vi "ACC_LabVIEW_Read_Example.vi"() -> ()   [LabVIEW 2014, in "ACC_LabVIEW.lvlib"]
doc: "Example for using the \"read\" method."
uses:
  ACC_LabVIEW.lvlib
  DataConverter/Acc2LabVIEWData_String.vi
  DataConverter/Acc2LabVIEWData_SWord.vi
panel:
  out "EFICD":T1
  out "LV_TimeStamp":T2
  out "Device Properties":T3(array[cluster])
  out "error out":errorcluster
  in  "#of expected Elements in \"Acc_Data_Out\"":u32=200
  in  "Propname[20]":string="PROPDESC"
  in  "Nomenklatur[6]":string="K4XCS012"
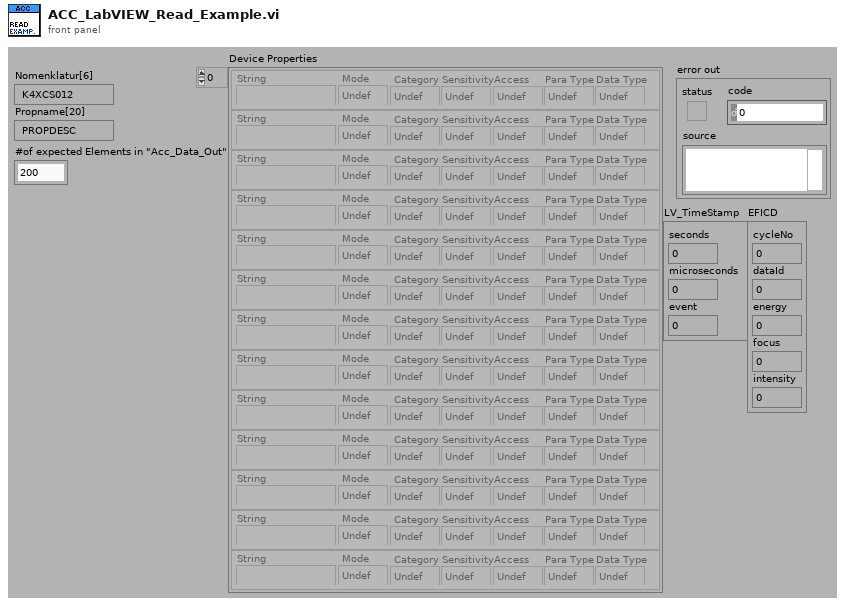
[diagram p1: front panel]
types:
  T1 = cluster{"cycleNo":u32, "dataId":u32, "energy":u32, "focus":u32, "intensity":u32}
  T2 = cluster{"seconds":u32, "microseconds":u32, "event":u32}
  T3 = cluster{"String":string, " Mode":enum16{"Undef", "Read", "Write", "Call"}, " Category":enum16{"Undef", "Master", "Slave"}, "Sensitivity":enum16{"Undef", "All", "VrtAcc", "None"}, "Access":enum16{"Undef", "Free", "Device", "System", "Critical"}, "Para Type":enum16{"Undef", "BitSet8", "BitSet16", "BitSet32", "Integer16", "Integer32", "Fix16", "Fix32", "RealF", "Real32", "Integer8", "RealG", "Structure", "BitSet64", "Integer64", "Real64"}, "Data Type":enum16{"Undef", "BitSet8", "BitSet16", "BitSet32", "Integer16", "Integer32", "Fix16", "Fix32", "RealF", "Real32", "Integer8", "RealG", "Structure", "BitSet64", "Integer64", "Real64"}}[]
  T4 = typedef "ACC_LabVIEW.lvlib/ACC_LabVIEW_Container.ctl" = cluster{"Data Type":T5, "String":string, "Double":dbl}
  T5 = typedef "ACC_LabVIEW.lvlib/ACC_LabVIEW_DataTypes.ctl" = enum16{"SByte (8Bit Int signed)", "UByte (8Bit int unsigned)", "SWord (16Bit Int signed)", "UWord (16Bit Int unsigned)", "SLong (32Bit Int signed)", "ULong (32Bit Int unsigned)", "Float32 (float)", "Float64 (double)", "String"}
  T6 = cluster{"Value":string, "Value":i16, "Value":i16, "Value":i16, "Value":i16, "Value":i16, "Value":i16}
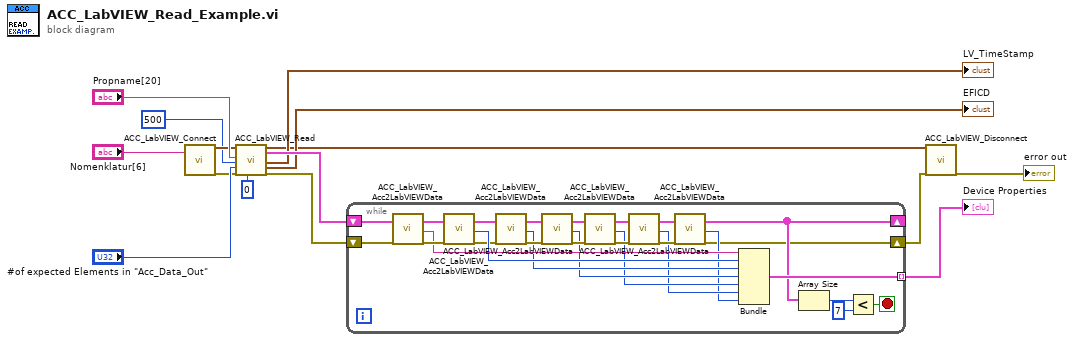
[diagram p0: block diagram]
diagram:
  n1 = call "ACC_LabVIEW_Connect.vi"("Nomenklatur"="Nomenklatur[6]") -> ("DeviceReferenceOut"=w5:cluster{"ID":u32}, "error out"=w8:errorcluster)  [unwired: 17 in]
  n2 = call "ACC_LabVIEW_Read.vi"("DeviceReferenceIn"=w5, "Propname"="Propname[20]", "return data string buffer size (Byte)"=u32 500 ("return strings buffer size (Byte)"), "#of expected Elements in \"Acc_Data_Out\""="#of expected Elements in \"Acc_Data_Out\"", "error in (no error)"=w8, "VirtAcc"=0) -> ("DeviceReferenceOut"=w7:cluster{"ID":u32}, "Acc_Data_Out"=w12:T4[], "LV_TimeStamp"=→"LV_TimeStamp":T2, "EFICD"=→"EFICD":T1, "error out"=w4:errorcluster)  [unwired: 9 in]
  n3 = while {
    shift-right: [w20] -> _
    shift-left: w12 -> [w41]
    tunnel: [w42] -> w9 mode=indexing
    shift-right: [w19] -> w6
    shift-left: w4 -> [w40]
    stop <- w16 stop-if-true
    n4 = call-poly "ACC_LabVIEW_Acc2LabVIEWData.vi"("Acc_Data_In"=w41, "error in"=w40) -> ("Acc_Data_Out"=w39:T4[], "Value"=w37:string, "error out"=w38:errorcluster)  [unwired: 15 in]
    n5 = call-poly "ACC_LabVIEW_Acc2LabVIEWData.vi"("Acc_Data_In"=w39, "error in"=w38) -> ("Acc_Data_Out"=w27:T4[], "Value"=w36:i16, "error out"=w26:errorcluster)  [unwired: 15 in]
    n6 = call-poly "ACC_LabVIEW_Acc2LabVIEWData.vi"("Acc_Data_In"=w27, "error in"=w26) -> ("Acc_Data_Out"=w35:T4[], "Value"=w25:i16, "error out"=w34:errorcluster)  [unwired: 15 in]
    n7 = call-poly "ACC_LabVIEW_Acc2LabVIEWData.vi"("Acc_Data_In"=w35, "error in"=w34) -> ("Acc_Data_Out"=w33:T4[], "Value"=w24:i16, "error out"=w32:errorcluster)  [unwired: 15 in]
    n8 = call-poly "ACC_LabVIEW_Acc2LabVIEWData.vi"("Acc_Data_In"=w33, "error in"=w32) -> ("Acc_Data_Out"=w29:T4[], "Value"=w23:i16, "error out"=w28:errorcluster)  [unwired: 15 in]
    n9 = call-poly "ACC_LabVIEW_Acc2LabVIEWData.vi"("Acc_Data_In"=w29, "error in"=w28) -> ("Acc_Data_Out"=w31:T4[], "Value"=w22:i16, "error out"=w30:errorcluster)  [unwired: 15 in]
    n10 = call-poly "ACC_LabVIEW_Acc2LabVIEWData.vi"("Acc_Data_In"=w31, "error in"=w30) -> ("Acc_Data_Out"=w20:T4[], "Value"=w21:i16, "error out"=w19:errorcluster)  [unwired: 15 in]
    n11 = Bundle("Value"=w37, "Value"=w36, "Value"=w25, "Value"=w24, "Value"=w23, "Value"=w22, "Value"=w21) -> (w42:T6)  [unwired: 1 in]
    n12 = Array Size(array=w20) -> (size(s)=w17:i32)
    n13 = Less?(x=w17, y=7) -> (x < y?=w16:bool)
  }
  "Device Properties" <- w9
  n14 = call "ACC_LabVIEW_Disconnect.vi"("DeviceReferenceIn"=w7, "error in (no error)"=w6) -> ("error out"=→"error out":errorcluster)  [unwired: 17 in]
